vi "DAQ.Auto Configure.vi"(8 "error in (no error)":errorcluster, 11 "Instrument.DAQ":refnum<class "Instrument.DAQ.lvclass">) -> (0 "error out":errorcluster, 3 "Instrument.DAQ out":refnum<class "Instrument.DAQ.lvclass">)   [LabVIEW 2019, in "Instrument.Lockin.lvlib" / "Instrument.DAQ.lvclass"]
uses:
  Instrument.DAQ.lvclass
  Instrument.DAQ.lvclass/Instrument.DAQ.ctl
  DAQmx/DAQmx.lvclass
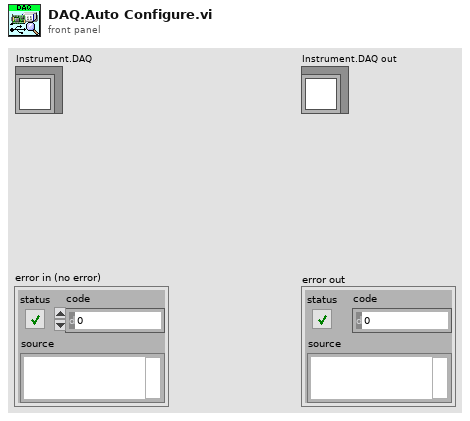
[diagram p1: front panel]
types:
  T1 = typedef "DAQmx.lvclass/DAQ.Config.AO--Cluster--Array.ctl" = T2[]
  T2 = typedef "DAQmx.lvclass/DAQ.Config.AO--Cluster.ctl" = cluster{"Channels":tag, "Range":T3, "output terminal configuration":i32, "Type":T4}
  T3 = typedef "DAQmx.lvclass/DAQ.Config.AO.Range--enum.ctl" = enum16{"±0.1", "±1.0", "±10.0", ""}
  T4 = typedef "DAQmx.lvclass/DAQ.Config.Device Type--enum.ctl" = enum16{"None", "USB-4431", "PXI-446x"}
  T5 = typedef "DAQmx.lvclass/DAQ.Config.AI--Cluster--Array.ctl" = T6[]
  T6 = typedef "DAQmx.lvclass/DAQ.Config.AI--Cluster.ctl" = cluster{"Channels":tag, "Coupling":T7, "Range":T8, "input terminal configuration":i32, "Type":T4}
  T7 = typedef "DAQmx.lvclass/DAQ.Config.AI.Coupling--enum.ctl" = u16
  T8 = typedef "DAQmx.lvclass/DAQ.Config.AI.Range--enum.ctl" = enum16{"±0.316", "±1.00", "±3.16", "±10.0", "±31.6", "±42.4", ""}
  T9 = typedef "DAQmx.lvclass/DeviceInfo--Cluster.ctl" = cluster{"DeviceName":string, "DevIsSimulated":bool, "DeviceSerialNumber":u32, "ProductType":string, "ProductCategory":i32, "ProductNumber":u32, "ChassisNumber":u32, "SlotNumber":u32, "ChassisName":string, "ChassisSerialNumber":u32}
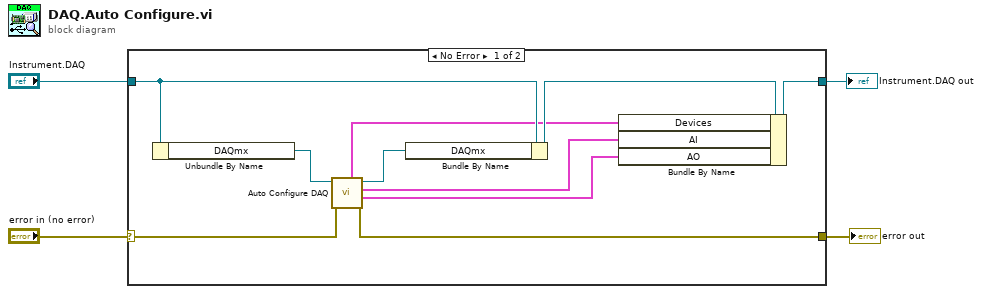
[diagram p0: block diagram]
diagram:
  n1 = case shown="No Error" "error in (no error)" {
    selector: "error in (no error)" -> [w8 w15]
    tunnel: [w5 w15] -> w4
    tunnel: "Instrument.DAQ" -> [w13 w16]
    tunnel: [w14 w16] -> w2
    frame No Error {
      n2 = Unbundle By Name(w13) -> ("DAQmx"=w7:refnum<class "DAQmx.lvclass">)
      n3 = call "Auto Configure DAQ.vi"("error in (no error)"=w8, "DAQmx in"=w7) -> ("error out"=w5:errorcluster, "Configuration.AO"=w10:T1, "Configuration.AI"=w11:T5, "DAQmx out"=w6:refnum<class "DAQmx.lvclass">, "Devices"=w9:T9[])  [unwired: 5 in]
      n4 = Bundle By Name(cluster=w13, "DAQmx"=w6) -> (w12:refnum<class "Instrument.DAQ.lvclass">)
      n5 = Bundle By Name(cluster=w12, "Devices"=w9, "AI"=w11, "AO"=w10) -> (w14:refnum<class "Instrument.DAQ.lvclass">)
    }
    frame Error {
    }
  }
  "error out" <- w4
  "Instrument.DAQ out" <- w2
